vi "Set_defaults.vi"(8 "error in":errorcluster, 11 "References In":T1) -> (0 "error out":errorcluster, 3 "References Out":T1)   [LabVIEW 2016]
uses:
  References.ctl
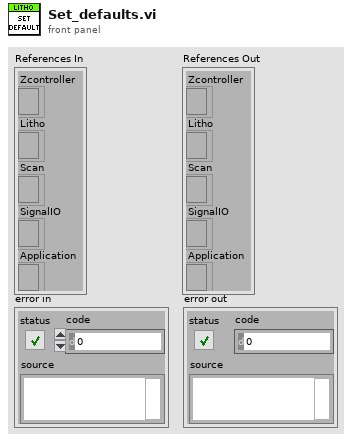
[diagram p1: front panel]
types:
  T1 = typedef "References.ctl" = cluster{"Zcontroller":refnum<k7>, "Litho":refnum<k7>, "Scan":refnum<k7>, "SignalIO":refnum<k7>, "Application":refnum<k7>}
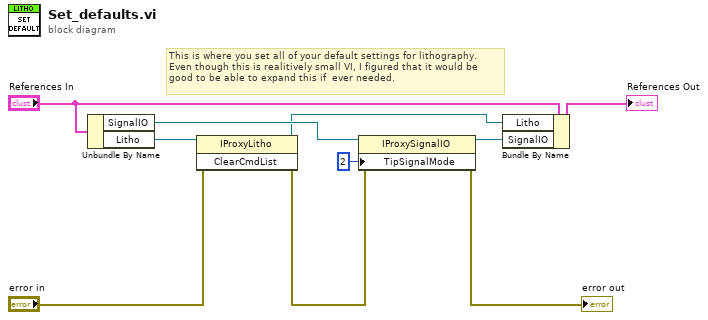
[diagram p0: block diagram]
diagram:
  # "This is where you set all of your default settings for lithography.\nEven though this is realitively small VI, I figured that it would be\ngood to be able to expand this if  ever needed."
  n1 = Unbundle By Name("References In") -> ("SignalIO"=w8:refnum<k7>, "Litho"=w10:refnum<k7>)
  n2 = invoke class="IProxyLitho" method="ClearCmdList"(reference=w10, error in="error in") -> (reference out=w3:refnum<k7>, error out=w9:errorcluster)  [unwired: 1 in, 1 out]
  n3 = property class="IProxySignalIO"(reference=w8, error in=w9, "TipSignalMode"=2) -> (reference out=w4:refnum<k7>, error out=→"error out":errorcluster)
  n4 = Bundle By Name(cluster="References In", "Litho"=w3, "SignalIO"=w4) -> (→"References Out":T1)
